vi "Write_waveform.vi"(8 "error in (no error)":errorcluster, 9 "operation (0:open)":T1(ring)=enum."replace or create", 10 "Array":dbl[](array[numeric]), 11 "Write_to_file in":refnum<class "Write_to_file.lvclass">) -> (0 "error out":errorcluster, 3 "Write_to_file out":refnum<class "Write_to_file.lvclass">)   [LabVIEW 2019, in "Write_to_file.lvclass"]
uses:
  Write_to_file.lvclass
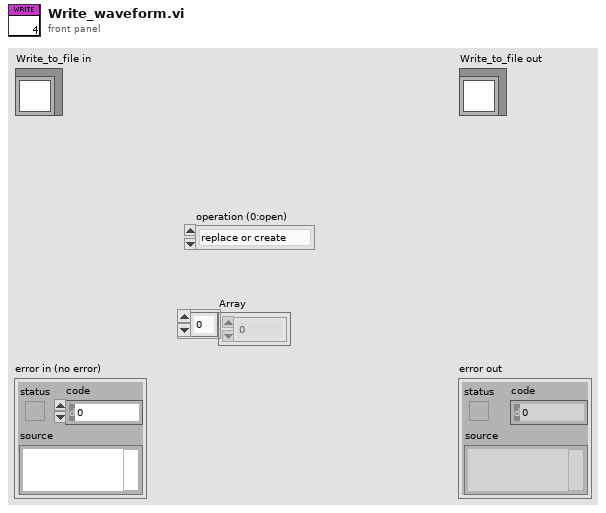
[diagram p1: front panel]
types:
  T1 = enum16{"open", "replace", "create", "open or create", "replace or create", "replace or create with confirmation"}
  T2 = enum16{"big-endian, network order", "native, host order", "little-endian"}
  T3 = enum16{"open", "open or create", "create or replace", "create", "open (read-only)"}
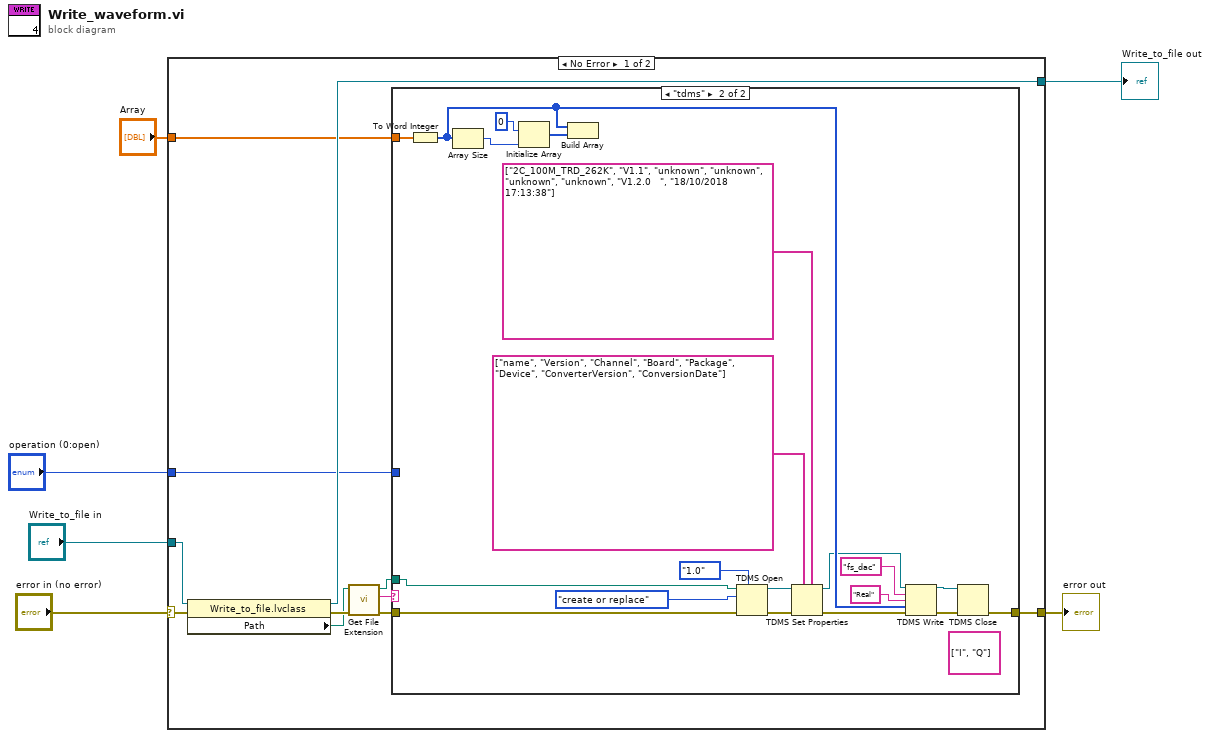
[diagram p0: block diagram]
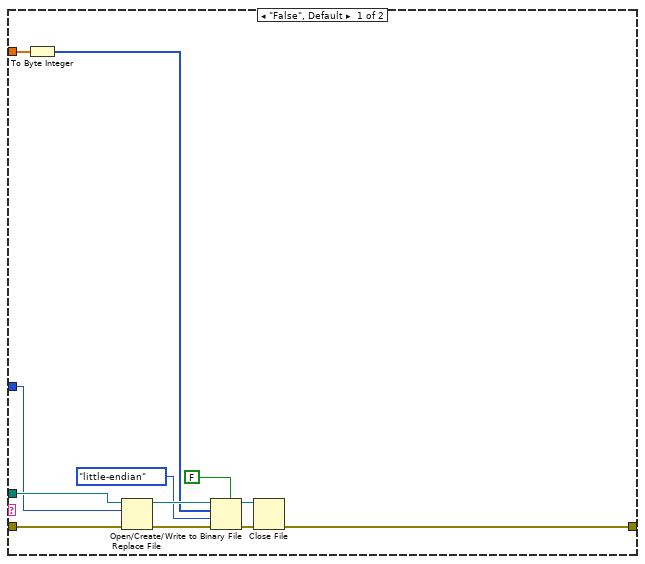
[diagram p2: hidden frame]
diagram:
  n1 = case shown="No Error" "error in (no error)" {
    selector: "error in (no error)" -> [w15 w51]
    tunnel: [w14 w51] -> w5
    tunnel: [w16 w50] -> w3
    tunnel: "Write_to_file in" -> [w17 w50]
    tunnel: "Array" -> [w13 _]
    tunnel: "operation (0:open)" -> [w12 _]
    frame No Error {
      n2 = property class="Write_to_file.lvclass"(reference=w17, error in=w15) -> (reference out=w16:refnum<class "Write_to_file.lvclass">, error out=w10:errorcluster, "Path"=w8:path)
      n3 = call <vilib>:"Get File Extension.vi"("error in (no error)"=w10, "file"=w8) -> ("error out"=w9:errorcluster, "lowercase file extension"=w11:string, "dup file"=w7:path)  [unwired: 5 in, 2 out]
      n4 = case shown="\"tdms\"" w11 {
        tunnel: w9 -> [w25 w49]
        tunnel: [w22 w40] -> w14
        tunnel: w7 -> [w21 w48]
        tunnel: w13 -> [w20 w45]
        tunnel: w12 -> [w19 _]
        frame "False", Default {
          n5 = To Byte Integer(number=w20) -> (8bit integer=w18:i8[])
          n6 = Open/Create/Replace File(file path (use dialog)=w21, error in=w25, operation (0:open)=w19) -> (refnum out=w29:refnum<file>, error out=w24:errorcluster)  [unwired: 3 in, 1 out]
          n7 = Write to Binary File(file (use dialog)=w29, data=w18, error in=w24, 5:FALSE ("prepend array or string size? (T)"), 9:T2."little-endian" ("byte order (0:big-endian, network order)")) -> (refnum out=w28:refnum<file>, error out=w23:errorcluster)  [unwired: 1 in, 1 out]
          n8 = Close File(refnum=w28, error in=w23) -> (error out=w22:errorcluster)  [unwired: 1 out]
        }
        frame "tdms" {
          (unwired) string[] ["I", "Q"] ("channel name(s) in (Untitled)")
          n9 = To Word Integer(number=w45) -> (16bit integer=w37:i16[])
          n10 = Array Size(array=w37) -> (size(s)=w38:i32)
          n11 = Initialize Array(i16 0, w38) -> (w44:i16[])
          n12 = Build Array(w37, w44) -> ()  [unwired: 1 out]
          n13 = TDMS Open(7:enum16{"1.0", "2.0"}."1.0" ("file format version (2.0)"), 8:w49, 10:T3."create or replace" ("operation (0:open)"), 11:w48) -> (0:w46:errorcluster, 3:w33:refnum<k34>)  [unwired: 3 in]
          n14 = TDMS Set Properties(5:string[] ["2C_100M_TRD_262K", "V1.1", "unknown", "unknown", "unknown", "unknown", "V1.2.0   ", "18/10/2018 17:13:38"] ("Values"), 7:string[] ["name", "Version", "Channel", "Board", "Package", "Device", "ConverterVersion", "ConversionDate"] ("property names"), 8:w46, 11:w33) -> (0:w34:errorcluster, 3:w32:refnum<k34>)  [unwired: 2 in, 2 out]
          n15 = TDMS Write(0:w32, 5:"fs_dac" ("group name in (Untitled)"), 7:"Real" ("group name in (Untitled)"), 9:w37, 11:w34) -> (4:w41:refnum<k34>, 15:w42:errorcluster)  [unwired: 1 in, 2 out]
          n16 = TDMS Close(8:w42, 11:w41) -> (0:w40:errorcluster)  [unwired: 1 out]
        }
      }
    }
    frame Error {
    }
  }
  "error out" <- w5
  "Write_to_file out" <- w3
